vi "ScopeInit.vi"(1 "error in (no error)":errorcluster) -> (0 "error out":errorcluster)   [LabVIEW 2018]
uses:
  <instrlib>/Tektronix DPO MSO 2000 4000 Series/Public/Configure/Configure Trigger (Edge).vi
  <instrlib>/Tektronix DPO MSO 2000 4000 Series/Tektronix DPO MSO 2000 4000 Series.lvlib
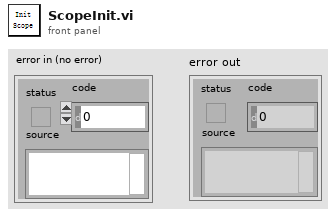
[diagram p1: front panel]
types:
  T1 = typedef "IMAQ Image.ctl" = refnum<image>
  T2 = cluster{"示波器":cluster{"Channel (0:Channel 1)":enum16{"Channel 1", "Channel 2", "Channel 3", "Channel 4"}, "电压范围":dbl, "触发电压":dbl, "时间范围":dbl, " 示波器VISA":refnum<visa-resource-name>, "时间范围 标签":u64, "电压范围 标签":u64, "触发电压 标签":u64}, "光谱仪":cluster{"Channel (0:Channel 1)":enum16{"Channel 1", "Channel 2", "Channel 3", "Channel 4"}, "电压范围":u64, "触发电压":u64, "时间范围":u64}, " 近场相机":cluster{"曝光时间":i32, "模拟增益":i32, "控制套接字":i32, "IP 地址":string, " 采集套接字":i32, "  版本号":i32, "ImageData":T1, "  增益最大":i32, "  增益最小":i32, " 曝光最大":i32, " 曝光最小":i32, " 帧速":i32, " 同步切换":i32, "  曝光缩放":i32}, " 偏振仪":cluster{"电压范围":u64, "触发电压":u64, "时间范围":u64, "波长范围":enum16{"可见光 400-700nm", "近红外 700-1100nm"}, "可见光偏振测量仪VISA":refnum<visa-resource-name>, "近红外偏振测量仪VISA":refnum<visa-resource-name>}, " 功率计":cluster{"通道":enum16{"Channel 1", "Channel 2"}, "工作波长":u32, "单位":u64, "时间范围":u64, "IP地址":string, "端口":u32}, "能量计":cluster{"通道":enum16{"Channel 1", "Channel 2"}, "工作波长":u32, "单位":u64, "时间范围":u64, "IP地址":string, "端口":u32, "能量计量程":enum16{"200uJ", "20uJ", "2uJ", "200nJ"}}, "电机":cluster{"Channel (0:Channel 1)":enum16{"Channel 1", "Channel 2", "Channel 3", "Channel 4"}, "电压范围":u64, "触发电压":u64, "时间范围":u64}, " 远场相机":cluster{"曝光时间":i32, "模拟增益":i32, "控制套接字":i32, "IP 地址":string, " 采集套接字":i32, "  版本号":i32, "ImageData":T1, "  增益最大":i32, "  增益最小":i32, " 曝光最大":i32, " 曝光最小":i32, " 帧速":i32, " 同步切换":i32, "  曝光缩放":i32}}
  T3 = cluster{"Channel (0:Channel 1)":enum16{"Channel 1", "Channel 2", "Channel 3", "Channel 4"}, "电压范围":dbl, "触发电压":dbl, "时间范围":dbl, " 示波器VISA":refnum<visa-resource-name>, "时间范围 标签":u64, "电压范围 标签":u64, "触发电压 标签":u64}
  T4 = enum16{"Channel 1", "Channel 2", "Channel 3", "Channel 4"}
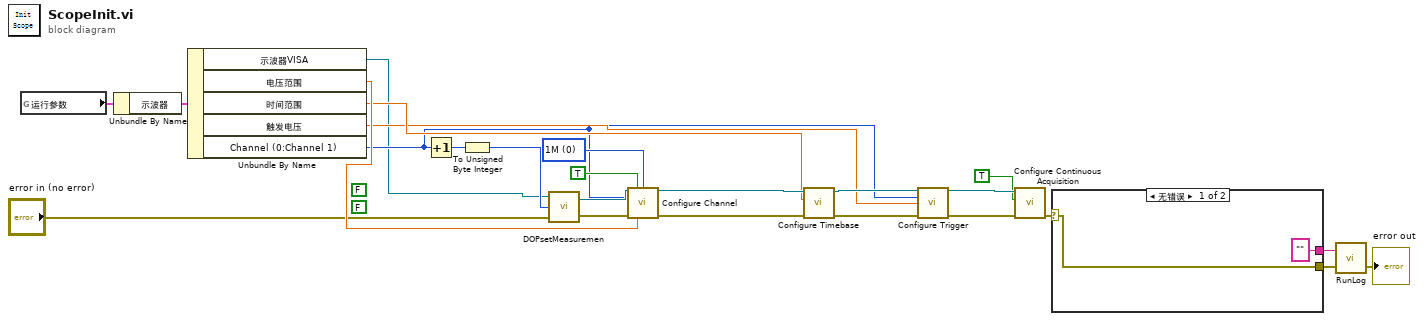
[diagram p0: block diagram]
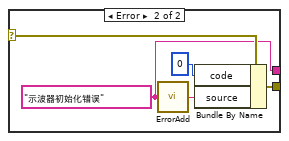
[diagram p2: hidden frame]
diagram:
  (unwired) FALSE ("Reset (True)")
  (unwired) FALSE ("ID Query (True)")
  w20 = u16 0 items=["1M", "75", "50"] ("Input Impedance (0: 1M ohm)")
  n1 = global read "参数.vi" "运行参数"() -> (w12:T2)
  n2 = Unbundle By Name(w12) -> ("示波器"=w11:T3)
  n3 = Unbundle By Name(w11) -> ("示波器VISA"=w2:refnum<visa-resource-name>, "电压范围"=w10:dbl, "时间范围"=w9:dbl, "触发电压"=w8:dbl, "Channel (0:Channel 1)"=w7:T4)
  n4 = Increment(x=w7) -> (x+1=w25:T4)
  n5 = To Unsigned Byte Integer(number=w25) -> (unsigned 8bit integer=w24:u8)
  n6 = call "DOPsetMeasuremen.vi"("error in (no error)"="error in (no error)", "CH"=w24, "VISA resource name"=w2) -> ("error out"=w22:errorcluster, "VISA resource name out"=w23:refnum<visa-resource-name>)
  n7 = call <instrlib>:"Configure Channel.vi"("VISA resource name"=w23, "Enable Channel (T: Enable)"=TRUE, "Input Impedance (0: 1M ohm)"=w20, "Channel (0: Channel 1)"=w7, "error in (no error)"=w22, "Vertical Range (10.0 V)"=w10) -> ("VISA resource name out"=w19:refnum<visa-resource-name>, "error out"=w18:errorcluster)  [unwired: 8 in]
  n8 = call <instrlib>:"Configure Timebase.vi"("error in (no error)"=w18, "Timebase (0.0005 s)"=w9, "VISA resource name"=w19) -> ("error out"=w16:errorcluster, "VISA resource name out"=w17:refnum<visa-resource-name>)  [unwired: 7 in]
  n9 = call-poly <instrlib>:"Configure Trigger.vi"("VISA resource name"=w17, "Trigger Source (0: Channel 1)"=w7, "Trigger Level (0.0 V)"=w8, "error in (no error)"=w16) -> ("VISA resource name out"=w15:refnum<visa-resource-name>, "error out"=w14:errorcluster)  [unwired: 10 in]
  n10 = call <instrlib>:"Configure Continuous Acquisition.vi"("error in (no error)"=w14, "Enable Continuous Acquisition Mode (T: Enable)"=TRUE, "VISA resource name"=w15) -> ("error out"=w6:errorcluster)  [unwired: 7 in, 1 out]
  n11 = case shown="无错误" w6 {
    selector: w6 -> [w27 w32]
    tunnel: [w27 w29] -> w5
    tunnel: ["" ("source") w28] -> w4
    frame No Error {
    }
    frame Error {
      w28 = "示波器初始化错误" ("source")
      n12 = call "ErrorAdd.vi"("source"=w28) -> ("Errorout Souce"=w30:string)
      n13 = Bundle By Name(cluster=w32, "code"=0, "source"=w30) -> (w29:errorcluster)
    }
  }
  n14 = call "RunLog.vi"("error in"=w5, "Message"=w4) -> ("error out"=→"error out":errorcluster)  [unwired: 1 in]
